vi "Matrix left divisionMM.vi"(2 "A":dbl[][](array[numeric]), 3 "number of iterations":i32=2, 4 "B":dbl[][](array[numeric]), 5 "SVD relative tolerance":dbl) -> (0 "error":i32, 1 "B\\A":dbl[][](array[numeric]))   [LabVIEW 2010, in "NI_Gmath.lvlib"]
doc: "Left division operator. B\\A solves the equation B*X=A. When used with two polynomials, \\ is overloaded to produce a transfer function whose numerator is the right-hand operand. When used with two dynamic systems, a new system is created whose state matrix is the appended states of the two systems and whose output matrix is that of the \"numerator\" system. (For systems in transfer- function format, the new system is obtained by multiplying the \"numerator\" system by the reciprocal of the \"denominator\" system.) For matrix division, there are no specific conditions on the dimensions of A and B but the condition of B affects the accuracy of the matrix quotient obtained. An error message appears if B is singular. If B is square and nonsingular, B\\A returns a matrix X with the same dimensions as A. An LU (Gaussian) decomposition, rather than a direct inverse, is used. If the condition estimate of B is less than the machine epsilon, a warning message appears. If B is non-square, X is the least-squares solution to B*X=A and has row dimension equal to the number of columns of B and column dimension equal to the number of columns of A. This operation uses a QR decomposition to implicitly compute the rank of B; the solution X will have no more nonzero components in each column than this rank value."
uses:
  NI_Gmath.lvlib
  Real SVD Decomposition.vi
  A x Vector.vi
  NI_AALBase.lvlib
  NI_AALPro.lvlib
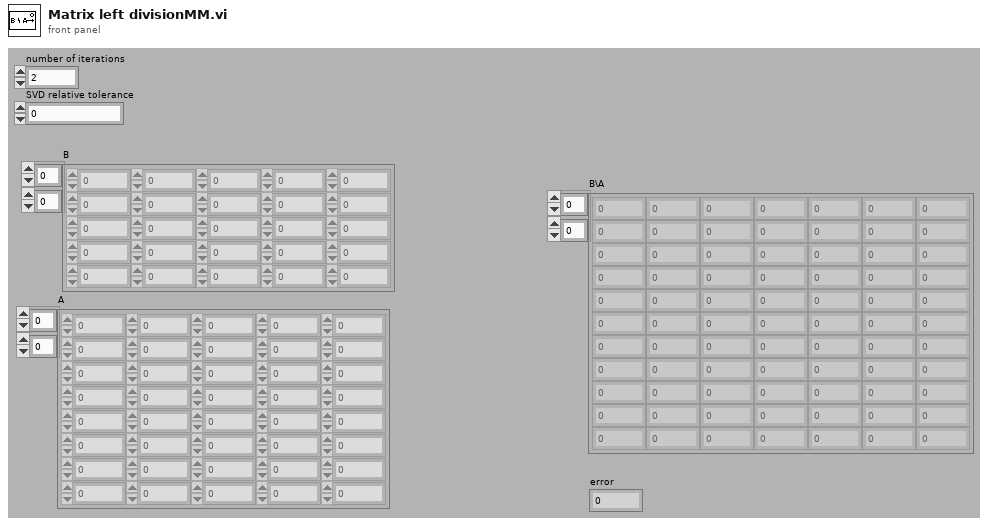
[diagram p1: front panel]
types:
  T1 = typedef "NI_Matrix.lvlib/RealMatrix.ctl" = dbl[][]
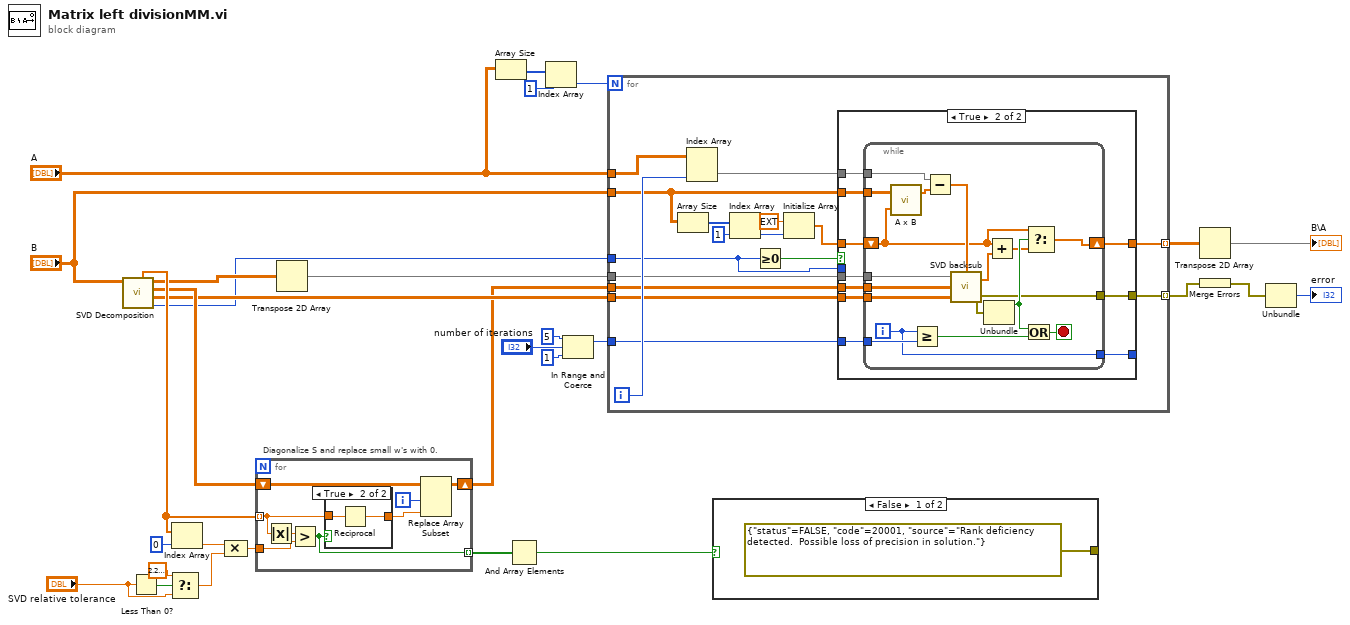
[diagram p0: block diagram]
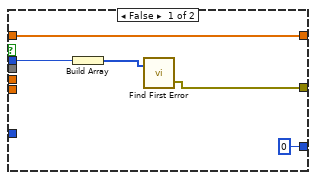
[diagram p2: hidden frame]
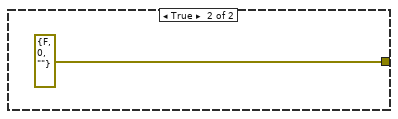
[diagram p3: hidden frame]
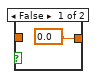
[diagram p4: hidden frame]
diagram:
  # "Diagonalize S and replace small w's with 0."
  n1 = call-poly "SVD Decomposition.vi"("A"="B") -> ("error"=w8:i32, "Matrix V"=w15:T1, "Matrix S"=w16:T1, "Matrix U"=w22:T1, "Vector S"=w23:dbl[])  [unwired: 6 in]
  n2 = Less Than 0?(x="SVD relative tolerance") -> (x < 0?=w21:bool)
  n3 = Select(t=2.220446049250313e-16, s=w21, f="SVD relative tolerance") -> (s? t:f=w19:dbl)
  n4 = Index Array(array=w23, index=0) -> (element=w25:dbl)
  n5 = Compound Arithmetic op=MULTIPLY(w25, w19) -> (w26:dbl)
  n6 = for {
    tunnel: w23 -> [w34] mode=indexing
    shift-right: [w37] -> w14
    shift-left: w16 -> [w36]
    tunnel: w26 -> [w32]
    tunnel: [w31] -> w18 mode=indexing
    i -> [w38]
    n7 = Absolute Value(x=w34) -> (abs(x)=w33:dbl)
    n8 = Greater?(x=w33, y=w32) -> (0:w31:bool)
    n9 = case shown="True" w31 {
      tunnel: w34 -> [_ w41]
      tunnel: [0.0 w40] -> w35
      frame False {
      }
      frame True {
        n10 = Reciprocal(x=w41) -> (1/x=w40:dbl)
      }
    }
    n11 = Replace Array Subset(array=w36, new element=w35, index (row)=w38, index (col)=w38) -> (w37:T1)
  }
  n12 = Transpose 2D Array(2D array=w22) -> (transposed array=w13:T1)
  n13 = Array Size(array="A") -> (size(s)=w4:i32[])
  n14 = And Array Elements(Boolean array=w18) -> (logical AND=w17:bool)
  n15 = Index Array(array=w4, index=1) -> (element=w2:i32)
  n16 = In Range and Coerce(upper limit=5, x="number of iterations", lower limit=1) -> (coerced(x)=w9:i32)  [unwired: 1 out]
  n17 = for {
    N: w2 -> [_]
    tunnel: w15 -> [w56]
    tunnel: w14 -> [w55]
    tunnel: w13 -> [w54]
    tunnel: [w53] -> w5 mode=indexing
    tunnel: w9 -> [w50]
    tunnel: w8 -> [w48]
    tunnel: "B" -> [w45]
    tunnel: "A" -> [w44]
    tunnel: [w43] -> w1 mode=indexing
    i -> [w58]
    n18 = Array Size(array=w45) -> (size(s)=w52:i32[])
    n19 = Index Array(array=w44, index (col)=w58) -> (element=w42:dbl[])  [unwired: 1 in]
    n20 = Index Array(array=w52, index=1) -> (element=w47:i32)
    n21 = Greater Or Equal To 0?(x=w48) -> (x >= 0?=w49:bool)
    n22 = Initialize Array(ext 0.0 ("element"), w47) -> (w57:ext[])
    n23 = case shown="True" w49 {
      tunnel: w45 -> [_ w73]
      tunnel: [w63 w72] -> w43
      tunnel: w57 -> [w63 w71]
      tunnel: w42 -> [_ w70]
      tunnel: w56 -> [_ w69]
      tunnel: w55 -> [_ w68]
      tunnel: w54 -> [_ w67]
      tunnel: w50 -> [_ w66]
      tunnel: [w60 w65] -> w53
      tunnel: [0 w64] -> _
      tunnel: w48 -> [w62 _]
      frame False {
        n24 = Build Array(w62) -> (w61:i32[])
        n25 = call "Find First Error.vi"("error codes"=w61) -> ("error out"=w60:errorcluster)  [unwired: 3 in, 1 out]
      }
      frame True {
        n26 = while {
          shift-right: [w79] -> w72
          shift-left: w71 -> [w78]
          tunnel: w73 -> [w90]
          tunnel: w70 -> [w76]
          tunnel: w67 -> [w88]
          tunnel: w68 -> [w87]
          tunnel: w69 -> [w86]
          tunnel: w66 -> [w84]
          tunnel: [w77] -> w65
          tunnel: [w74] -> w64
          i -> [w74]
          stop <- w82 stop-if-true
          n27 = call-poly "A x B.vi"("Vector"=w78, "A"=w90) -> ("A x Vector"=w75:dbl[])  [unwired: 1 out]
          n28 = Greater Or Equal?(x=w74, y=w84) -> (x >= y?=w83:bool)
          n29 = Subtract ("Subtract.vi")(x=w76, y=w75) -> (x-y=w85:dbl[])
          n30 = call "SVD backsub.vi"("A"=w85, "V"=w86, "1/S"=w87, "U^T"=w88) -> ("error out"=w77:errorcluster, "solution"=w89:dbl[])
          n31 = Unbundle(w77) -> ("status"=w81:bool)  [unwired: 2 out]
          n32 = Add(x=w78, y=w89) -> (x+y=w80:ext[])
          n33 = Or(x=w81, y=w83) -> (x .or. y?=w82:bool)
          n34 = Select(t=w78, s=w81, f=w80) -> (s? t:f=w79:ext[])
        }
      }
    }
  }
  n35 = case shown="False" w17 {
    tunnel: [errorcluster {"status"=FALSE, "code"=20001, "source"="Rank deficiency detected.  Possible loss of precision in solution."} ("error out") errorcluster {"status"=FALSE, "code"=0, "source"=""} ("error out")] -> _
    frame False {
    }
    frame True {
    }
  }
  n36 = Transpose 2D Array(2D array=w1) -> (transposed array=→"B\\A":ext[][])
  n37 = Merge Errors(w5) -> (w7:errorcluster)
  n38 = Unbundle(w7) -> ("code"=→"error":i32)  [unwired: 2 out]
